vi "PCO_GetFlimMasterModulationFrequency.vi"(8 "error in (no error)":errorcluster {"code" format="%x"}, 11 "ph":u64) -> (0 "error out":errorcluster {"code" format="%x"}, 1 "dwFrequency":u32, 2 "ErrorMessage":i32 format="%x", 3 "ph out":u64)   [LabVIEW 2019, in "SDK.lvlib" / "SpecialCommandsFlim.lvlib"]
doc: "<b>Description:</b>\nThis function can be used to query the current modulation frequency, which is used when the camera is configured as frequency master (see function PCO_SetFlimModulationParameter).\n\n<b>Supported camera type</b>\npco.flim\n\n<b>Descriptor dependency:</b>\nNone"
uses:
  SpecialCommandsFlim.lvlib
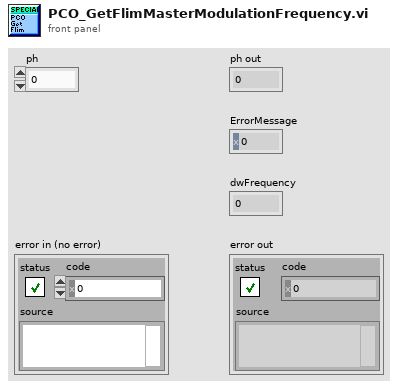
[diagram p1: front panel]
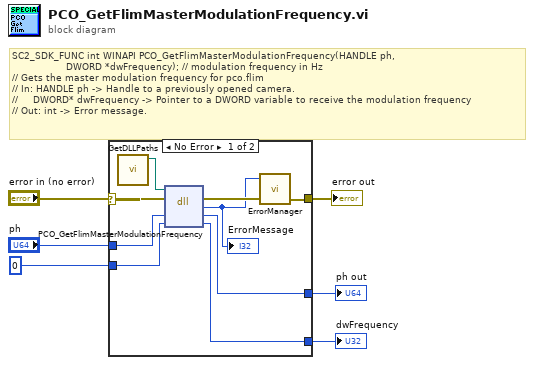
[diagram p0: block diagram]
diagram:
  # "SC2_SDK_FUNC int WINAPI PCO_GetFlimMasterModulationFrequency(HANDLE ph, \n                  DWORD *dwFrequency); // modulation frequency in Hz\n// Gets the master modulation frequency for pco.flim\n// In: HANDLE ph -> Handle to a previously opened camera.\n//     DWORD* dwFrequency -> Pointer to a DWORD variable to receive the modulation frequency\n// Out: int -> Error message."
  n1 = case shown="No Error" "error in (no error)" {
    selector: "error in (no error)" -> [w11 w18]
    tunnel: "ph" -> [w15 w17]
    tunnel: [w14 w17] -> w5
    tunnel: u32 0 ("dwFrequency") -> [w13 w16]
    tunnel: [w12 w16] -> w3
    tunnel: [w10 w18] -> w2
    frame No Error {
      n2 = call "GetDLLPaths.vi"() -> ("SC2_Cam_Path"=w7:path)  [unwired: 8 in, 3 out]
      n3 = dll-call lib="?" fn="PCO_GetFlimMasterModulationFrequency"(path in=w7, error in=w11, "ph"=w15, "dwFrequency"=w13) -> (error out=w9:errorcluster, "return type"=w8:i32, "ph"=w14:u64, "dwFrequency"=w12:u32)  [unwired: 1 in, 1 out]
      "ErrorMessage" <- w8
      n4 = call "ErrorManager.vi"("error in (no error)"=w9, "error code"=w8) -> ("error out"=w10:errorcluster)  [unwired: 2 in, 1 out]
    }
    frame Error {
    }
  }
  "ph out" <- w5
  "dwFrequency" <- w3
  "error out" <- w2
